vi "Create DI Channel.vi"(6 "index":i32, 8 "error in":errorcluster, 9 "default value":bool, 10 "name":string, 11 "DI channel in":refnum<class "DI Channel.lvclass">) -> (0 "error out":errorcluster, 3 "DI channel out":refnum<class "DI Channel.lvclass">)   [LabVIEW 2020, in "Scan Engine Scripting.lvlib" / "DI Channel.lvclass"]
uses:
  DI Channel.lvclass
  Channel/Type.ctl
  Channel/Channel.lvclass
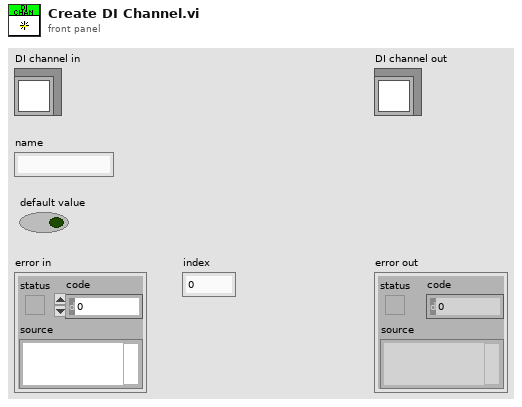
[diagram p1: front panel]
types:
  T1 = typedef "Scan Engine Scripting.lvlib/Channel.lvclass/Type.ctl" = enum16{"Input", "Output"}
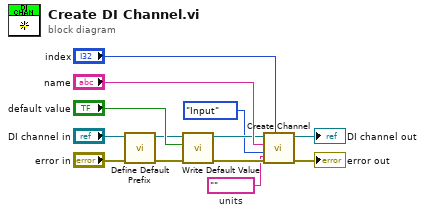
[diagram p0: block diagram]
diagram:
  w1 = ""  # units
  n1 = call-dynamic "Define Default Prefix.vi"("error in"="error in", "DI channel in"="DI channel in") -> ("error out"=w2:errorcluster, "DI channel out"=w4:refnum<class "DI Channel.lvclass">)  [unwired: 8 in]
  n2 = call-dynamic "Write Default Value.vi"("error in"=w2, "default value"="default value", "digital channel in"=w4) -> ("error out"=w12:errorcluster, "digital channel out"=w10:refnum<class "DI Channel.lvclass">)  [unwired: 7 in]
  n3 = call-dynamic "Create Channel.vi"("units"=w1, "index"="index", "error in"=w12, "type"=Type."Input", "name"="name", "channel in"=w10) -> ("error out"=→"error out":errorcluster, "channel out"=→"DI channel out":refnum<class "DI Channel.lvclass">)  [unwired: 4 in]
